vi "trigger_start.vi"(10 "Trigger source in":tag="/cDAQ4/PFI0", 11 "Trigger counter":tag="cDAQ4/_ctr0") -> (0 "error out":errorcluster, 2 "Trigger source out":tag, 3 "Refnum out":refnum<k21>)   [LabVIEW 2022 SP3]
uses:
  <vilib>/DAQmx/create/channels.llb/DAQmx Create Channel (CO-Pulse Generation-Time).vi
  <vilib>/DAQmx/configure/trigger.llb/DAQmx Start Trigger (Digital Edge).vi
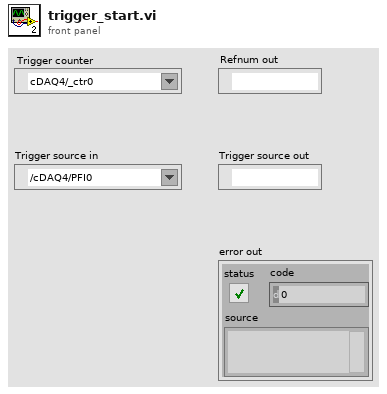
[diagram p1: front panel]
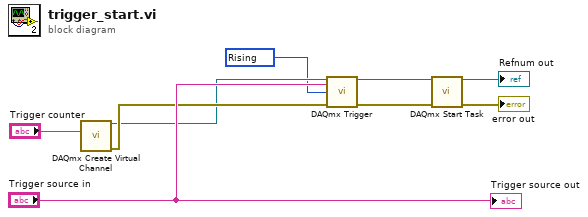
[diagram p0: block diagram]
diagram:
  w4 = 10280 items=["Rising"=10280, "Falling"=10171] ("edge")
  n1 = call-poly <vilib>:"DAQmx Create Virtual Channel.vi"("counter"="Trigger counter") -> ("task out"=w5:refnum<k21>, "error out"=w6:errorcluster)  [unwired: 13 in]
  n2 = call-poly <vilib>:"DAQmx Trigger.vi"("task/channels in"=w5, "source"="Trigger source in", "edge"=w4, "error in"=w6) -> ("task out"=w2:refnum<k21>, "error out"=w3:errorcluster)  [unwired: 10 in]
  n3 = call <vilib>:"DAQmx Start Task.vi"("task/channels in"=w2, "error in"=w3) -> ("task out"=→"Refnum out":refnum<k21>, "error out"=→"error out":errorcluster)  [unwired: 12 in]
  "Trigger source out" <- "Trigger source in"
